vi "Add Pending Transfer.vi"(8 "error in":errorcluster, 10 "SDO Transfer":refnum<class "SDO Transfer.lvclass">, 11 "Pending Transfers":refnum<data-value>) -> (0 "error out":errorcluster)   [LabVIEW 2020, in "CANopen.lvlib" / "SDO Manager.lvlib" / "SDO Manager.lvclass"]
uses:
  SDO Manager.lvclass
  SDO Transfer/SDO Transfer.lvclass
  SDO Transfer/SDO Transfer.lvclass/SDO Transfer.ctl
  SDO Manager.lvclass/SDO Manager.ctl
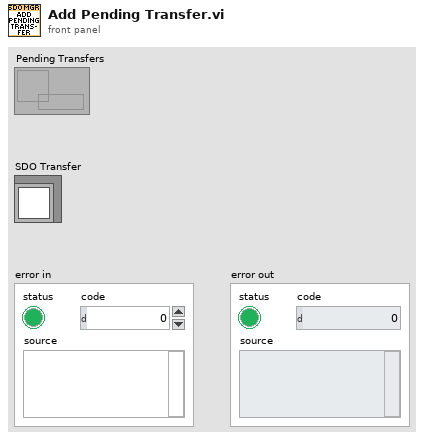
[diagram p1: front panel]
types:
  T1 = map{string, refnum<class "SDO Transfer.lvclass">}
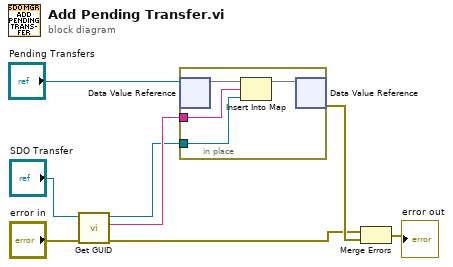
[diagram p0: block diagram]
diagram:
  n1 = call "Get GUID.vi"("error in"="error in", "SDO Transfer in"="SDO Transfer") -> ("error out"=w4:errorcluster, "GUID"=w2:string, "SDO Transfer out"=w1:refnum<class "SDO Transfer.lvclass">)  [unwired: 7 in]
  n2 = in-place {
    in-place-border: w1 -> [w10]
    in-place-border: w2 -> [w9]
    n3 = in-place-dvr #1("Pending Transfers") -> (w12:T1)  [unwired: 1 out]
    n4 = Insert Into Map(map in=w12, key=w9, value=w10) -> (map out=w11:T1)  [unwired: 2 out]
    n5 = in-place-dvr #1(w11) -> (w7:errorcluster)  [unwired: 1 out]
  }
  n6 = Merge Errors(w4, w7) -> (→"error out":errorcluster)
